vi "TDT-Get Events.vi"(0 "Data":T1={"TTankX"=refnum, "TDevAccX"=refnum, "LastTime"=0.0, "error"={"status"=FALSE, "code"=0, "source"=""}, "Block Name"="", "Circuit Tag"="", "Tank Name"="", "NumTicks"=0, "LastTick"=0.0, "Idle?"=FALSE, "Wait (ms)"=1000, "LastArtf"=0.0, "LastTosc"=0.0}, 11 "error in (no error)":errorcluster, 13 "Tetrode":bool) -> (4 "Data out":T1={"TTankX"=refnum, "TDevAccX"=refnum, "LastTime"=0.0, "error"={"status"=FALSE, "code"=0, "source"=""}, "Block Name"="", "Circuit Tag"="", "Tank Name"="", "NumTicks"=0, "LastTick"=0.0, "Idle?"=FALSE, "Wait (ms)"=1000, "LastArtf"=0.0, "LastTosc"=0.0}, 8 "Events":dbl[][](array[numeric]), 15 "error out":errorcluster)   [LabVIEW 2015]
uses:
  TDT Interface Data.ctl
panel:
  in  "Max Read":i32=20000
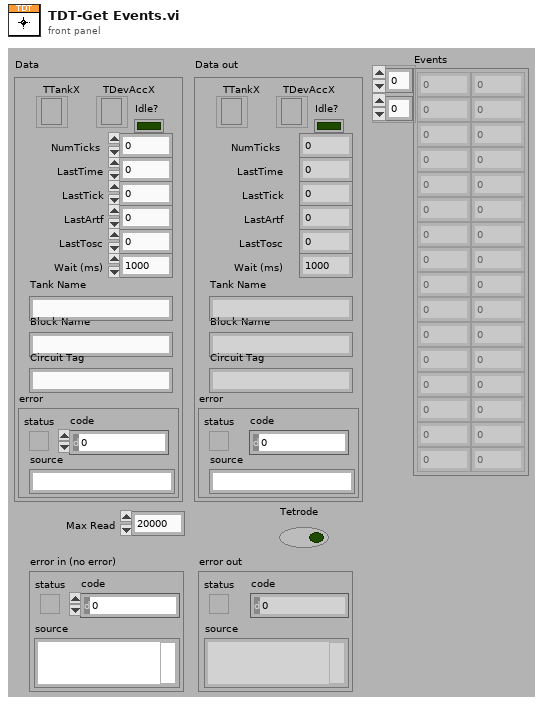
[diagram p1: front panel]
types:
  T1 = typedef "TDT Interface Data.ctl" = cluster{"TTankX":refnum<k7>, "TDevAccX":refnum<k7>, "LastTime":dbl, "error":errorcluster, "Block Name":string, "Circuit Tag":string, "Tank Name":string, "NumTicks":i32, "LastTick":dbl, "Idle?":bool, "Wait (ms)":u32, "LastArtf":dbl, "LastTosc":dbl}
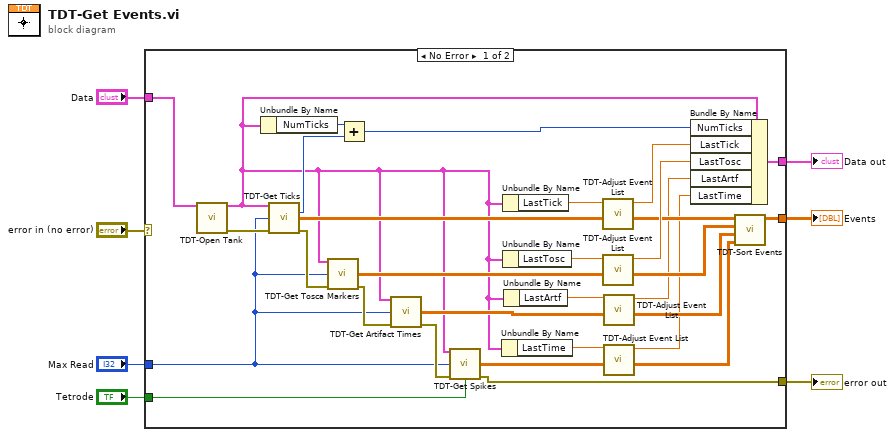
[diagram p0: block diagram]
diagram:
  n1 = case shown="No Error" "error in (no error)" {
    selector: "error in (no error)" -> [_ w39]
    tunnel: [w9 w39] -> w6
    tunnel: "Data" -> [w22 w38]
    tunnel: "Max Read" -> [w11 _]
    tunnel: [w26 _] -> w3
    tunnel: [w34 w38] -> w2
    tunnel: "Tetrode" -> [w8 _]
    frame No Error {
      n2 = call "TDT-Open Tank.vi"("Data"=w22) -> ("Data (out)"=w10:T1, "error out"=w23:errorcluster)  [unwired: 13 in]
      n3 = Unbundle By Name(w10) -> ("NumTicks"=w36:i32)
      n4 = call "TDT-Get Ticks.vi"("Data"=w10, "Max Read"=w11, "error in (no error)"=w23) -> ("Number of Ticks"=w35:i32, "Tick times"=w30:dbl[][], "error out"=w37:errorcluster)  [unwired: 9 in, 1 out]
      n5 = call "TDT-Get Tosca Markers.vi"("Data"=w10, "Max Read"=w11, "error in (no error)"=w37) -> ("Tosca markers"=w29:dbl[][], "error out"=w21:errorcluster)  [unwired: 10 in, 1 out]
      n6 = Add(x=w36, y=w35) -> (x+y=w33:i32)
      n7 = call "TDT-Get Artifact Times.vi"("Data"=w10, "Max Read"=w11, "error in (no error)"=w21) -> ("Artifact Times"=w20:dbl[][], "error out"=w12:errorcluster)  [unwired: 10 in, 1 out]
      n8 = call "TDT-Get Spikes.vi"("Data"=w10, "Max Read"=w11, "error in (no error)"=w12, "Tetrode"=w8) -> ("Spike times"=w13:dbl[][], "error out"=w9:errorcluster)  [unwired: 8 in, 2 out]
      n9 = Unbundle By Name(w10) -> ("LastTime"=w14:dbl)
      n10 = Unbundle By Name(w10) -> ("LastTick"=w32:dbl)
      n11 = Unbundle By Name(w10) -> ("LastTosc"=w28:dbl)
      n12 = Unbundle By Name(w10) -> ("LastArtf"=w19:dbl)
      n13 = call "TDT-Adjust Event List.vi"("Events in"=w30, "Last In"=w32) -> ("Events out"=w25:dbl[][], "Last out"=w31:dbl)  [unwired: 8 in]
      n14 = call "TDT-Adjust Event List.vi"("Events in"=w29, "Last In"=w28) -> ("Events out"=w24:dbl[][], "Last out"=w27:dbl)  [unwired: 8 in]
      n15 = call "TDT-Adjust Event List.vi"("Events in"=w20, "Last In"=w19) -> ("Events out"=w17:dbl[][], "Last out"=w18:dbl)  [unwired: 8 in]
      n16 = call "TDT-Adjust Event List.vi"("Events in"=w13, "Last In"=w14) -> ("Events out"=w16:dbl[][], "Last out"=w15:dbl)  [unwired: 8 in]
      n17 = Bundle By Name(cluster=w10, "NumTicks"=w33, "LastTick"=w31, "LastTosc"=w27, "LastArtf"=w18, "LastTime"=w15) -> (w34:T1)
      n18 = call "TDT-Sort Events.vi"("Tosca Markers"=w16, "Artifacts"=w17, "Spikes"=w24, "Ticks"=w25) -> ("Sorted events"=w26:dbl[][])  [unwired: 7 in]
    }
    frame Error {
    }
  }
  "error out" <- w6
  "Data out" <- w2
  "Events" <- w3
